vi "TestVI.vi"() -> ()   [LabVIEW 2010]
uses:
  <vilib>/Platform/NI_3dgraph.lvlib
  TypeDefs/ParameterCluster.ctl
panel:
  out "Waveform Graph 2":dbl[](graph)
  in  "3D Curve":refnum<k7>(container)
  out "Waveform Graph":dbl[](graph)
  out "size(s)":i32[](array[numeric])
  out "XY Point coordinates (um)":dbl[][](array[numeric])
  out "XY Graph":T1(graph)
  in  "Parameters":T2={"number of planes"=4, "z step"=1.9999999999999998e-05, "pixel dwell time"=1.0000000000000001e-11, "z frequency"=10.0, "number of pixels"=100, "smooth points"=10, "smooth line"=10, "Sine\nSawtooth"=FALSE, "PointSorting"=0, "Sort Points"=FALSE, "X-pixels"=256.0, "Y-lines"=256.0, "pixelstoµm"=256.0, "zoom"=1.0, "Time offset"=1.0000000000000001e-11} {"zoom" min=0.5 step=0.1; "Y-lines" min=1 step=1; "X-pixels" min=1 step=1; "PointSorting" items=["No Difference", "Every Second Point", "Down / Up"]; "smooth line" min=1; "smooth points" min=1; "number of pixels" min=1; "z frequency" format="%_4g"; "number of planes" min=1}
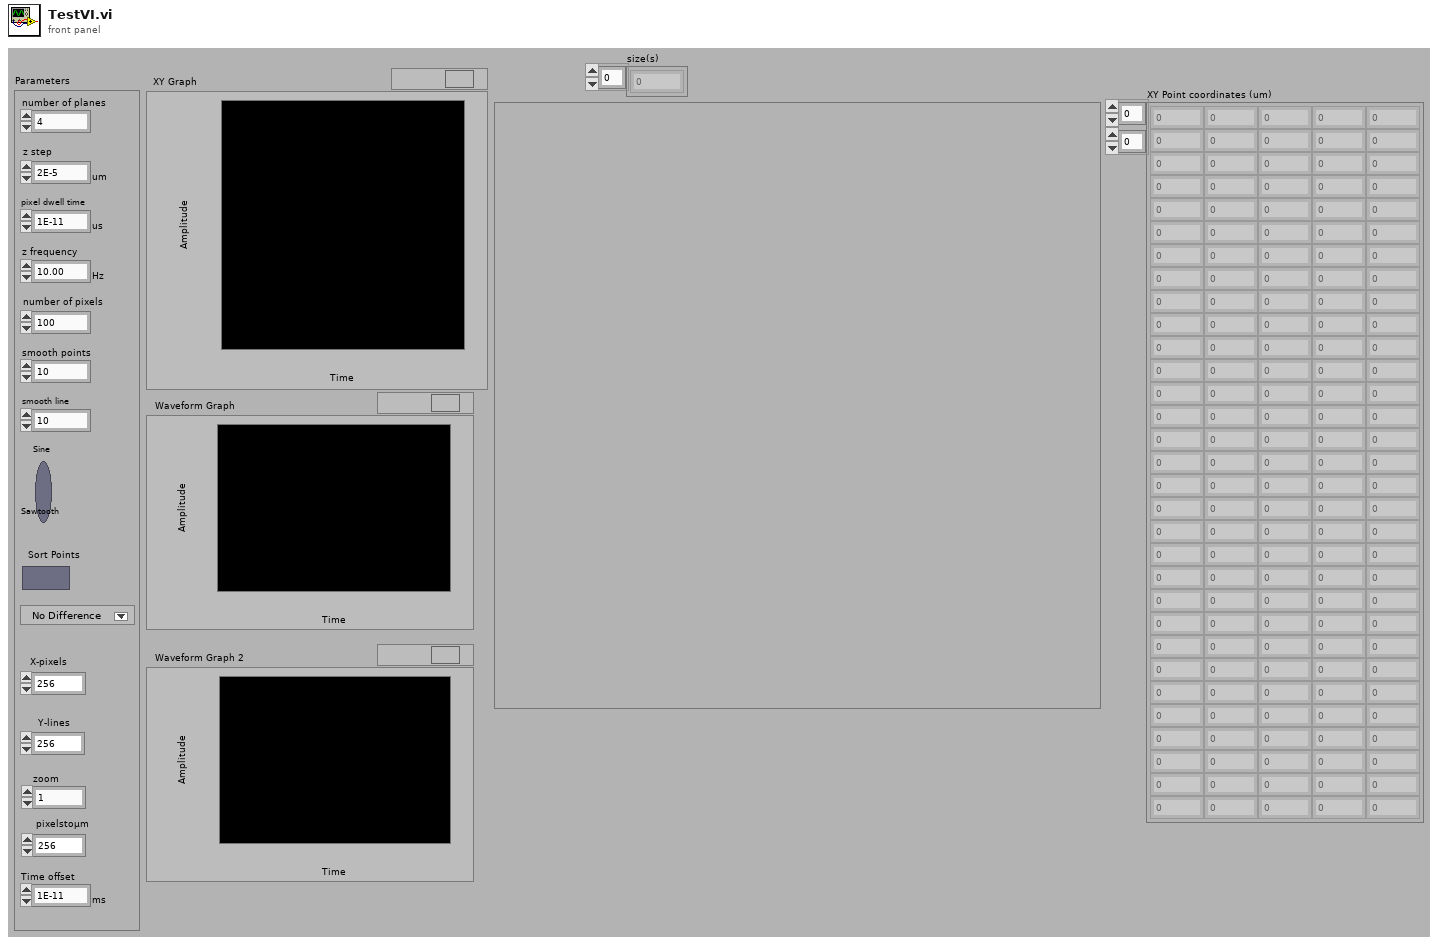
[diagram p1: front panel]
types:
  T1 = cluster{"x (pixels), y (pixels), z (um), time (s)":dbl[], "x (pixels), y (pixels), z (um), time (s)":dbl[]}
  T2 = typedef "ParameterCluster.ctl" = cluster{"number of planes":i32, "z step":dbl[unit], "pixel dwell time":dbl[unit], "z frequency":dbl[unit], "number of pixels":i32, "smooth points":i32, "smooth line":i32, "Sine\nSawtooth":bool, "PointSorting":u16, "Sort Points":bool, "X-pixels":sgl, "Y-lines":sgl, "pixelstoµm":dbl, "zoom":dbl, "Time offset":dbl[unit]}
  T3 = typedef "DutyCluster.ctl" = cluster{"points per plane":i32[], "NumberOfPoints":i32[], "number of planes to scan":i32, "Smooth":i32, "Points":dbl[][], "2*pi*f":dbl[unit], "period (s)":dbl[unit], "Amplitude":dbl[unit], "pixel length (um)":dbl[unit], "Time":dbl[unit][], "Signal":dbl[unit][], "Iteration":u16, "scan":i32[], "pause scanners":i32[], "Error?":bool, "Points on single plane":dbl[][][], "# of points on single plane":i32[], "scan offset z":i32, "min index":i32}
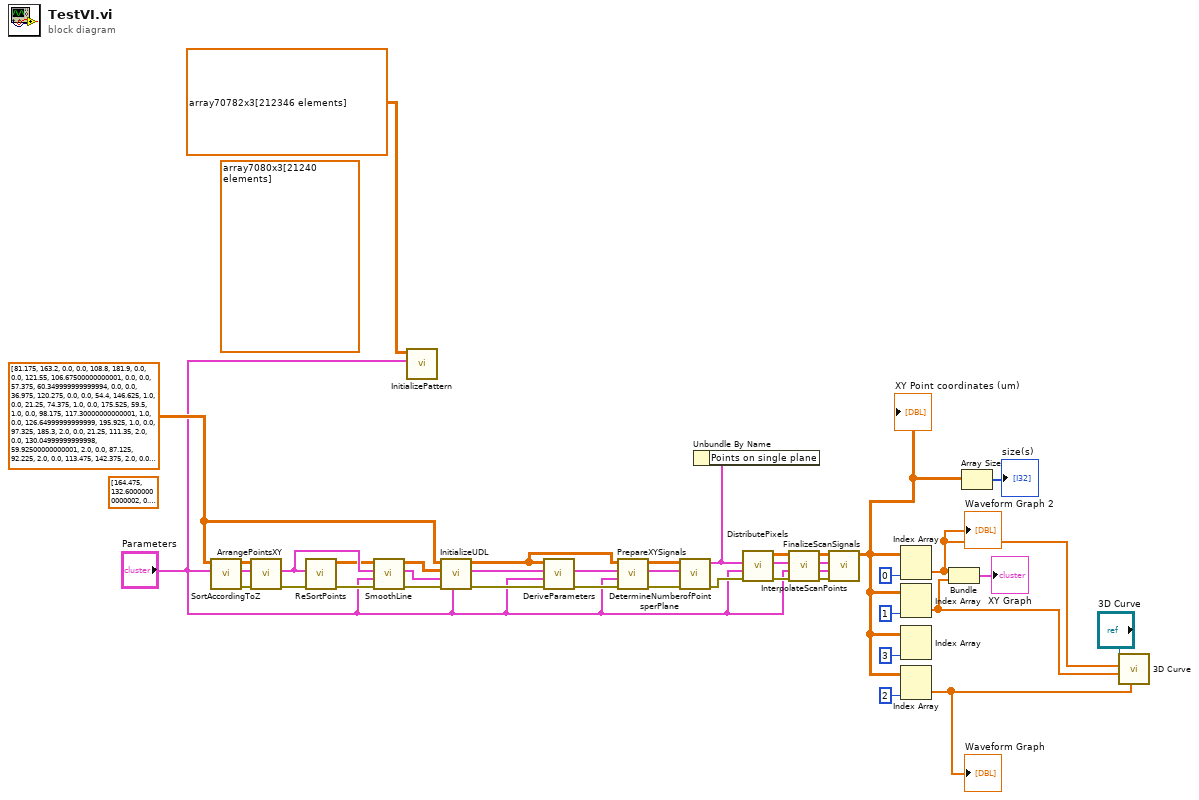
[diagram p0: block diagram]
diagram:
  w10 = dbl[][] [[81.175, 163.2, 0.0, 0.0], [108.8, 181.9, 0.0, 0.0], [121.55, 106.67500000000001, 0.0, 0.0], [57.375, 60.349999999999994, 0.0, 0.0], [36.975, 120.275, 0.0, 0.0], [54.4, 146.625, 1.0, 0.0], [21.25, 74.375, 1.0, 0.0], [175.525, 59.5, 1.0, 0.0], [98.175, 117.30000000000001, 1.0, 0.0], [126.64999999999999, 195.925, 1.0, 0.0], [97.325, 185.3, 2.0, 0.0], [21.25, 111.35, 2.0, 0.0], [130.04999999999998, 59.92500000000001, 2.0, 0.0], [87.125, 92.225, 2.0, 0.0], [113.475, 142.375, 2.0, 0.0], [72.675, 178.5, 3.0, 0.0], [13.6, 90.95000000000002, 3.0, 0.0], [143.225, 72.25, 3.0, 0.0], [83.725, 103.70000000000002, 3.0, 0.0], [105.825, 170.85000000000002, 3.0, 0.0]] ("subarray")
  (unwired) dbl[][] array7080x3[21240 elements] ("Pattern")
  (unwired) dbl[][] [[164.475, 132.60000000000002, 0.0, 0.0], [144.075, 187.85000000000002, 0.0, 0.0], [95.625, 160.22500000000002, 0.0, 0.0], [67.575, 82.875, 0.0, 0.0], [148.325, 70.125, 0.0, 0.0], [102.425, 119.85, 0.0, 0.0], [135.575, 170.425, 1.0, 0.0], [62.05, 143.65, 1.0, 0.0], [73.1, 87.975, 1.0, 0.0], [182.75, 72.67500000000001, 1.0, 0.0], [109.64999999999999, 127.925, 1.0, 0.0], [172.54999999999998, 170.425, 1.0, 0.0], [116.02499999999999, 180.625, 2.0, 0.0], [45.9, 125.80000000000001, 2.0, 0.0], [134.29999999999998, 85.85, 2.0, 0.0], [112.2, 125.375, 2.0, 0.0], [160.65, 164.05, 2.0, 0.0], [140.67499999999998, 228.225, 2.0, 0.0], [90.1, 174.25, 3.0, 0.0], [42.925, 101.15, 3.0, 0.0], [164.9, 80.75, 3.0, 0.0], [108.8, 116.025, 3.0, 0.0], [158.1, 159.8, 3.0, 0.0], [116.875, 214.2, 3.0, 0.0]] ("subarray")
  n1 = call "SortAccordingToZ.vi"("Parameters"="Parameters", "XYZ Point coordinates (pixels)"=w10) -> ("error out"=w41:errorcluster, "DutyCluster"=w40:T3, "XYZ Point coordinates updated (pixels)"=w8:dbl[][])  [unwired: 1 in, 6 out]
  n2 = call "ArrangePointsXY.vi"("error in (no error)"=w41, "DutyCluster"=w40, "XYZ Point coordinates (pixels)"=w8) -> ("error out"=w39:errorcluster, "DutyCluster"=w37:T3)  [unwired: 7 out]
  n3 = call "ReSortPoints.vi"("error in (no error)"=w39, "DutyCluster"=w37) -> ("error out"=w38:errorcluster, "Point coordinates resorte (pixels)"=w7:dbl[][])  [unwired: 1 in, 7 out]
  n4 = call "SmoothLine.vi"("error in (no error)"=w38, "Parameters"="Parameters", "DutyCluster"=w37, "XYZ Point coordinates (pixels)"=w7) -> ("error out"=w36:errorcluster, "DutyCluster"=w21:T3, "XYZ Point coordinates smoothed (pixels)"=w6:dbl[][])  [unwired: 5 out]
  n5 = call "InitializePattern.vi"("Parameters"="Parameters", "XYZ Point coordinates Pattern (pixels)"=dbl[][] array70782x3[212346 elements] ("Pattern")) -> ()  [unwired: 1 in, 9 out]
  n6 = call "InitializeUDL.vi"("Parameters"="Parameters", "error in (no error)"=w36, "DutyCluster"=w21, "XYZ Point coordinates smoothed (pixels)"=w6, "XYZ Point coordinates selected (pixels)"=w10) -> ("error out"=w35:errorcluster, "DutyCluster"=w3:T3, "XYZ Point coordinates (um)"=w4:dbl[][])  [unwired: 4 out]
  n7 = call "DeriveParameters.vi"("error in (no error)"=w35, "Parameters"="Parameters", "DutyCluster"=w3, "XYZ Point coordinates (pixels)"=w4) -> ("error out"=w34:errorcluster, "DutyCluster"=w20:T3)  [unwired: 6 out]
  n8 = call "PrepareXYSignals.vi"("error in (no error)"=w34, "Parameters"="Parameters", "DutyCluster"=w20, "XYZ Point coordinates (pixels)"=w4) -> ("error out"=w32:errorcluster, "DutyCluster"=w19:T3, "XY Point coordinates (um)"=w13:dbl[][])  [unwired: 5 out]
  n9 = call "DetermineNumberofPointsperPlane.vi"("error in (no error)"=w32, "DutyCluster"=w19, "XY coordinates (um)"=w13) -> ("error out"=w33:errorcluster, "DutyCluster"=w18:T3)  [unwired: 7 out]
  n10 = Unbundle By Name(w18) -> ()  [unwired: 1 out]
  n11 = call "DistributePixels.vi"("error in (no error)"=w33, "Parameters"="Parameters", "DutyCluster"=w18) -> ("error out"=w30:errorcluster, "DutyCluster"=w31:T3, "x pixels, y pixels, z, time"=w12:dbl[][])  [unwired: 6 out]
  n12 = call "InterpolateScanPoints.vi"("error in (no error)"=w30, "Parameters"="Parameters", "DutyCluster"=w31, "x pixels, y pixels, z, time"=w12) -> ("error out"=w27:errorcluster, "Parameters"=w28:T2, "DutyCluster"=w29:T3, "x pixels, y pixels, z, time"=w11:dbl[][])  [unwired: 4 out]
  n13 = call "FinalizeScanSignals.vi"("error in (no error)"=w27, "Parameters"=w28, "DutyCluster"=w29, "x pixels, y pixels, z, time"=w11) -> ("x (pixels), y (pixels), z (um), time (s)"=w5:dbl[][])  [unwired: 7 out]
  "XY Point coordinates (um)" <- w5
  n14 = Index Array(array=w5, index (col)=0 ("disabled index (col)")) -> (element=w14:dbl[])  [unwired: 1 in]
  "Waveform Graph 2" <- w14
  n15 = Index Array(array=w5, index (col)=1 ("disabled index (col)")) -> (element=w15:dbl[])  [unwired: 1 in]
  n16 = Index Array(array=w5, index (col)=3 ("disabled index (col)")) -> ()  [unwired: 1 in, 1 out]
  n17 = Index Array(array=w5, index (col)=2 ("disabled index (col)")) -> (element=w1:dbl[])  [unwired: 1 in]
  "Waveform Graph" <- w1
  n18 = Bundle("x (pixels), y (pixels), z (um), time (s)"=w14, "x (pixels), y (pixels), z (um), time (s)"=w15) -> (→"XY Graph":T1)  [unwired: 1 out]
  n19 = Array Size(array=w5) -> (size(s)=→"size(s)":i32[])
  n20 = call <vilib>:"3D Curve.vi"("z vector"=w1, "y vector"=w15, "x vector"=w14, "3D graph"="3D Curve") -> ()  [unwired: 1 in, 7 out]
